vi "Recursive File List.vi"(4 "Folders to Exclude":string[](array[string]), 6 "pattern":string, 8 "error in (no error)":errorcluster, 9 "Continue Recursing on Error? (F)":bool, 10 "Treat LLBs as Folders?":bool, 11 "Folder Path":path) -> (0 "error out":errorcluster, 1 "Number of Files":i32, 2 "All Files in Dir":path[](array[path]), 3 "dup Folder Path":path, 5 "All Folders":path[](array[path]))   [LabVIEW 2014]
doc: "Lists the contents of a folder or LLB."
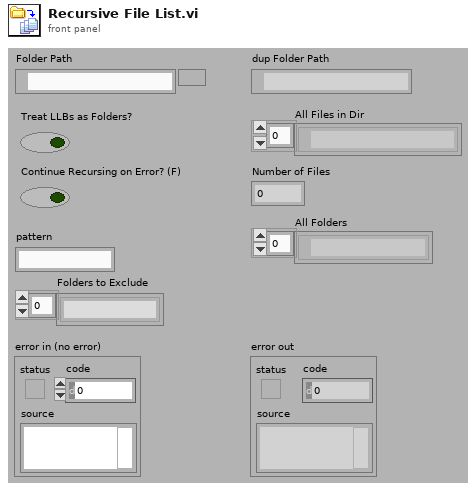
[diagram p1: front panel]
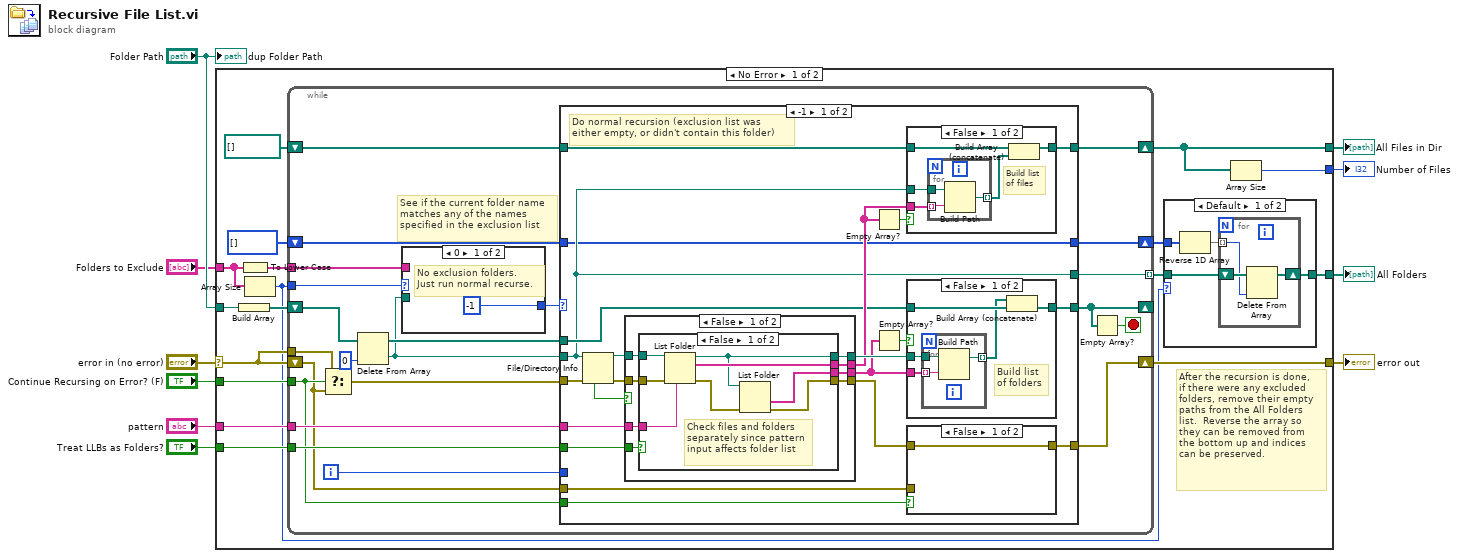
[diagram p0: block diagram]
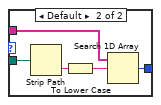
[diagram p3: hidden frame]
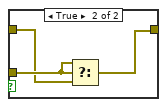
[diagram p5: hidden frame]
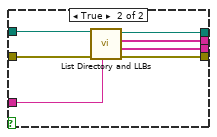
[diagram p6: hidden frame]
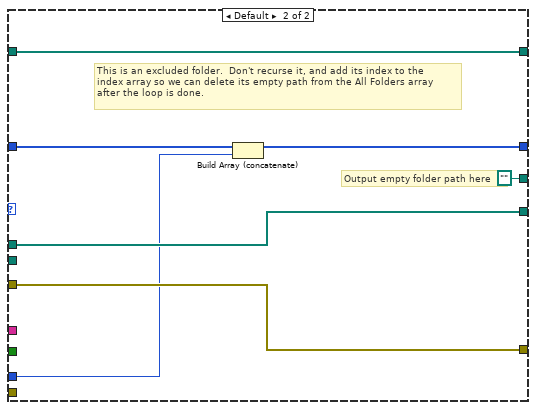
[diagram p9: hidden frame]
diagram:
  n1 = case shown="No Error" "error in (no error)" {
    selector: "error in (no error)" -> [w18 w139]
    tunnel: "Folder Path" -> [w27 _]
    tunnel: [w21 _] -> w10
    tunnel: [w20 _] -> w9
    tunnel: [w22 w139] -> w8
    tunnel: "Treat LLBs as Folders?" -> [w24 _]
    tunnel: [w12 _] -> w5
    tunnel: "pattern" -> [w23 _]
    tunnel: "Continue Recursing on Error? (F)" -> [w19 _]
    tunnel: "Folders to Exclude" -> [w15 _]
    frame No Error {
      # "After the recursion is done,\nif there were any excluded\nfolders, remove their empty\npaths from the All Folders\nlist.  Reverse the array so\nthey can be removed from\nthe bottom up and indices\ncan be preserved."
      n2 = Build Array(w27) -> (w26:path[])
      n3 = To Lower Case(string=w15) -> (all lower case string=w17:string[])
      n4 = Array Size(array=w15) -> (size(s)=w13:i32)
      n5 = while {
        shift-left: path[] [] ("Array Constant") -> [w55]
        shift-right: [w57] -> w21
        shift-left: w26 -> [w56]
        shift-right: [w52] -> _
        shift-right: [w46] -> w22
        shift-left: w18 -> [w45]
        tunnel: w24 -> [w54]
        tunnel: [w42] -> w14 mode=indexing
        tunnel: w23 -> [w53]
        tunnel: w19 -> [w47]
        tunnel: w18 -> [w48]
        tunnel: w17 -> [w38]
        shift-right: [w41] -> w11
        shift-left: i32[] [] -> [w43]
        tunnel: w13 -> [w39]
        i -> [w40]
        stop <- w51 stop-if-true
        # "See if the current folder name\nmatches any of the names\nspecified in the exclusion list"
        n6 = Select(t=w48, s=w47, f=w45) -> (s? t:f=w49:errorcluster)
        n7 = Delete From Array(array=w56, index=0) -> (deleted portion=w37:path, array with subset deleted=w44:path[])  [unwired: 1 in]
        n8 = case shown="0" w39 {
          tunnel: w38 -> [_ w60]
          tunnel: w37 -> [_ w63]
          tunnel: [-1 ("index of element") w59] -> w36
          frame 0 {
            # "No exclusion folders.\nJust run normal recurse."
          }
          frame Default {
            n9 = Strip Path(path=w63) -> (name=w62:string)  [unwired: 1 out]
            n10 = To Lower Case(string=w62) -> (all lower case string=w61:string)
            n11 = Search 1D Array(1D array=w60, element=w61) -> (index of element=w59:i32)  [unwired: 1 out]
          }
        }
        n12 = case shown="-1" w36 {
          tunnel: [w84 w138] -> w57
          tunnel: w55 -> [w83 w138]
          tunnel: w54 -> [w81 _]
          tunnel: w53 -> [w80 _]
          tunnel: [w77 w137] -> w52
          tunnel: w37 -> [w65 _]
          tunnel: w49 -> [w73 w136]
          tunnel: w47 -> [w71 _]
          tunnel: [w70 w136] -> w46
          tunnel: w45 -> [w69 _]
          tunnel: w44 -> [w66 w137]
          tunnel: w43 -> [w64 w135]
          tunnel: [w65 path ""] -> w42
          tunnel: [w64 w134] -> w41
          tunnel: w40 -> [_ w133]
          frame -1 {
            # "Do normal recursion (exclusion list was\neither empty, or didn't contain this folder)"
            n13 = File/Directory Info(path=w65, error in=w73) -> (path out=w75:path, error out=w76:errorcluster, shortcut=w74:bool)  [unwired: 4 out]
            n14 = case shown="False" w74 {
              tunnel: [w105 _] -> w67
              tunnel: [w104 w122] -> w82
              tunnel: [w103 w121] -> w72
              tunnel: w81 -> [w102 _]
              tunnel: w80 -> [w101 _]
              tunnel: [w100 _] -> w79
              tunnel: w76 -> [w99 w121]
              tunnel: w75 -> [w98 w122]
              frame False {
                n15 = case shown="False" w102 {
                  tunnel: [w113 w117] -> w105
                  tunnel: [w107 w116] -> w100
                  tunnel: w98 -> [w112 w120]
                  tunnel: [w106 w118] -> w104
                  tunnel: [w108 w115] -> w103
                  tunnel: w99 -> [w111 w119]
                  tunnel: w101 -> [w110 w114]
                  frame False {
                    # "Check files and folders\nseparately since pattern\ninput affects folder list"
                    n16 = List Folder(path=w112, pattern=w110, error in=w111) -> (path out=w106:path, filenames=w113:string[], error out=w109:errorcluster)  [unwired: 2 out]
                    n17 = List Folder(path=w106, error in=w109) -> (folder names=w107:string[], error out=w108:errorcluster)  [unwired: 4 out]
                  }
                  frame True {
                    n18 = call "List Directory and LLBs.vi"("pattern"=w114, "error in (no error)"=w119, "Folder Path"=w120) -> ("error out"=w115:errorcluster, "Folders and LLBs"=w116:string[], "Files sans LLBs"=w117:string[], "dup Folder Path"=w118:path)  [unwired: 5 out]
                  }
                }
              }
              frame True {
                # "Do not attempt to recurse the contents\nof folder shortcuts"
              }
            }
            n19 = Empty Array?(array=w67) -> (empty?=w68:bool)
            n20 = Empty Array?(array=w79) -> (empty?=w78:bool)
            n21 = case shown="False" w68 {
              tunnel: [w89 w93] -> w84
              tunnel: w67 -> [w88 _]
              tunnel: w83 -> [w87 w93]
              tunnel: w65 -> [w85 _]
              frame False {
                # "Build list of files"
                n22 = for {
                  tunnel: w88 -> [w91] mode=indexing
                  tunnel: w85 -> [w92]
                  tunnel: [w90] -> w86 mode=indexing
                  n23 = Build Path(base path=w92, name or relative path=w91) -> (appended path=w90:path)
                }
                n24 = Build Array (concatenate)(w87, w86) -> (w89:path[])
              }
              frame True {
              }
            }
            n25 = case shown="False" w78 {
              tunnel: w66 -> [w125 w131]
              tunnel: [w126 w131] -> w77
              tunnel: w82 -> [w127 _]
              tunnel: w79 -> [w123 _]
              frame False {
                # "Build list\nof folders"
                n26 = for {
                  tunnel: w127 -> [w130]
                  tunnel: [w129] -> w124 mode=indexing
                  tunnel: w123 -> [w128] mode=indexing
                  n27 = Build Path(base path=w130, name or relative path=w128) -> (appended path=w129:path)
                }
                n28 = Build Array (concatenate)(w124, w125) -> (w126:path[])
              }
              frame True {
              }
            }
            n29 = case shown="False" w71 {
              tunnel: w72 -> [w94 w96]
              tunnel: [w94 w95] -> w70
              tunnel: w69 -> [_ w97]
              frame False {
              }
              frame True {
                n30 = Select(t=w97, s=w97, f=w96) -> (s? t:f=w95:errorcluster)
              }
            }
          }
          frame Default {
            # "Output empty folder path here"
            # "This is an excluded folder.  Don't recurse it, and add its index to the\nindex array so we can delete its empty path from the All Folders array\nafter the loop is done."
            n31 = Build Array (concatenate)(w135, w133) -> (w134:i32[])
          }
        }
        n32 = Empty Array?(array=w52) -> (empty?=w51:bool)
      }
      n33 = case shown="Default" w13 {
        tunnel: w14 -> [w30 w35]
        tunnel: [w29 w35] -> w12
        tunnel: w11 -> [w31 _]
        frame Default {
          n34 = Reverse 1D Array(array=w31) -> (reversed array=w28:i32[])
          n35 = for {
            shift-right: [w33] -> w29
            shift-left: w30 -> [w34]
            tunnel: w28 -> [w32] mode=indexing
            n36 = Delete From Array(array=w34, index=w32) -> (array with subset deleted=w33:path[])  [unwired: 1 in, 1 out]
          }
        }
        frame 0 {
          # "No excluded folders.\nDon't run the code that\ndeletes excluded folder\nindices."
        }
      }
      n37 = Array Size(array=w21) -> (size(s)=w20:i32)
    }
    frame Error {
    }
  }
  "All Files in Dir" <- w10
  "Number of Files" <- w9
  "error out" <- w8
  "All Folders" <- w5
  "dup Folder Path" <- "Folder Path"
